vi "FPGA tester without DG535 settings.vi"() -> ()   [LabVIEW 2013]
uses:
  <vilib>/DAQmx/write.llb/DAQmx Write (Digital Bool 1Line 1Point).vi
  <vilib>/DAQmx/read.llb/DAQmx Read (Digital Bool 1Line 1Point).vi
  <vilib>/Utility/file.llb/Read From Spreadsheet File (I64).vi
  <vilib>/DAQmx/miscellaneous.llb/DAQmx Fill In Error Info.vi
panel:
  in  "Delay":u32
  out "Error out":errorcluster[][](array[cluster])
  in  "error in":errorcluster
  out "all rows":i64[][](array[numeric])
  in  "Read Excel file?":bool
  out "Current level":u16
  in  "Repetitions":dbl=1.0
  in  "Levels":i16[](array[numeric])
  out "Set 1":bool[](array[boolean])
  out "Set 2":bool[](array[boolean])
  out "Set 3":bool[](array[boolean])
  out "Set 4":bool[](array[boolean])
  out "16-bit number":bool[](array[boolean])
  # "Or specify levels below:"
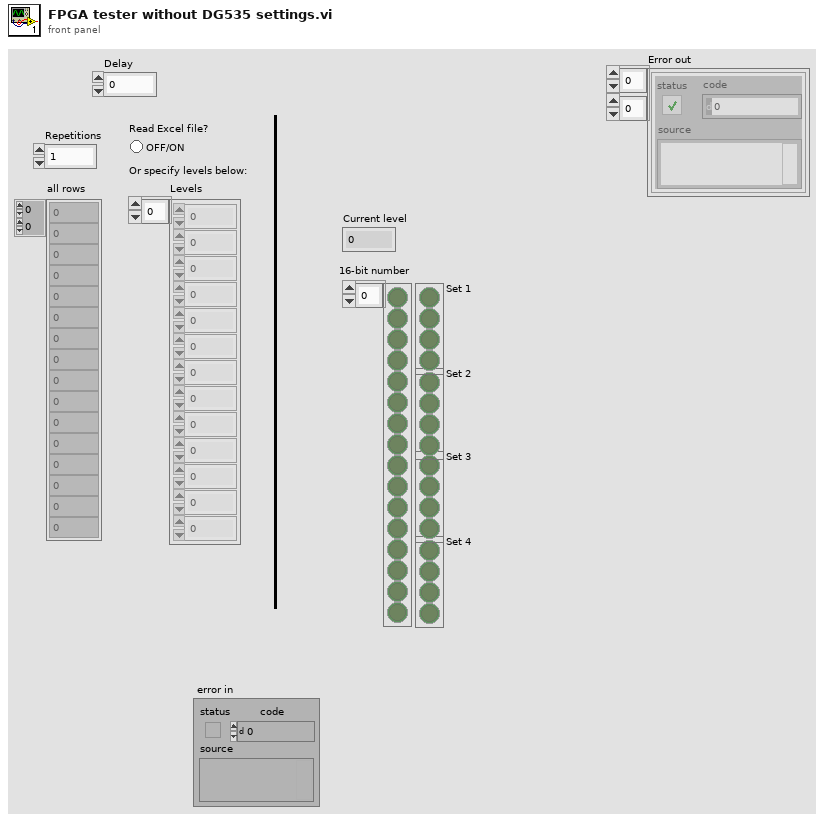
[diagram p1: front panel]
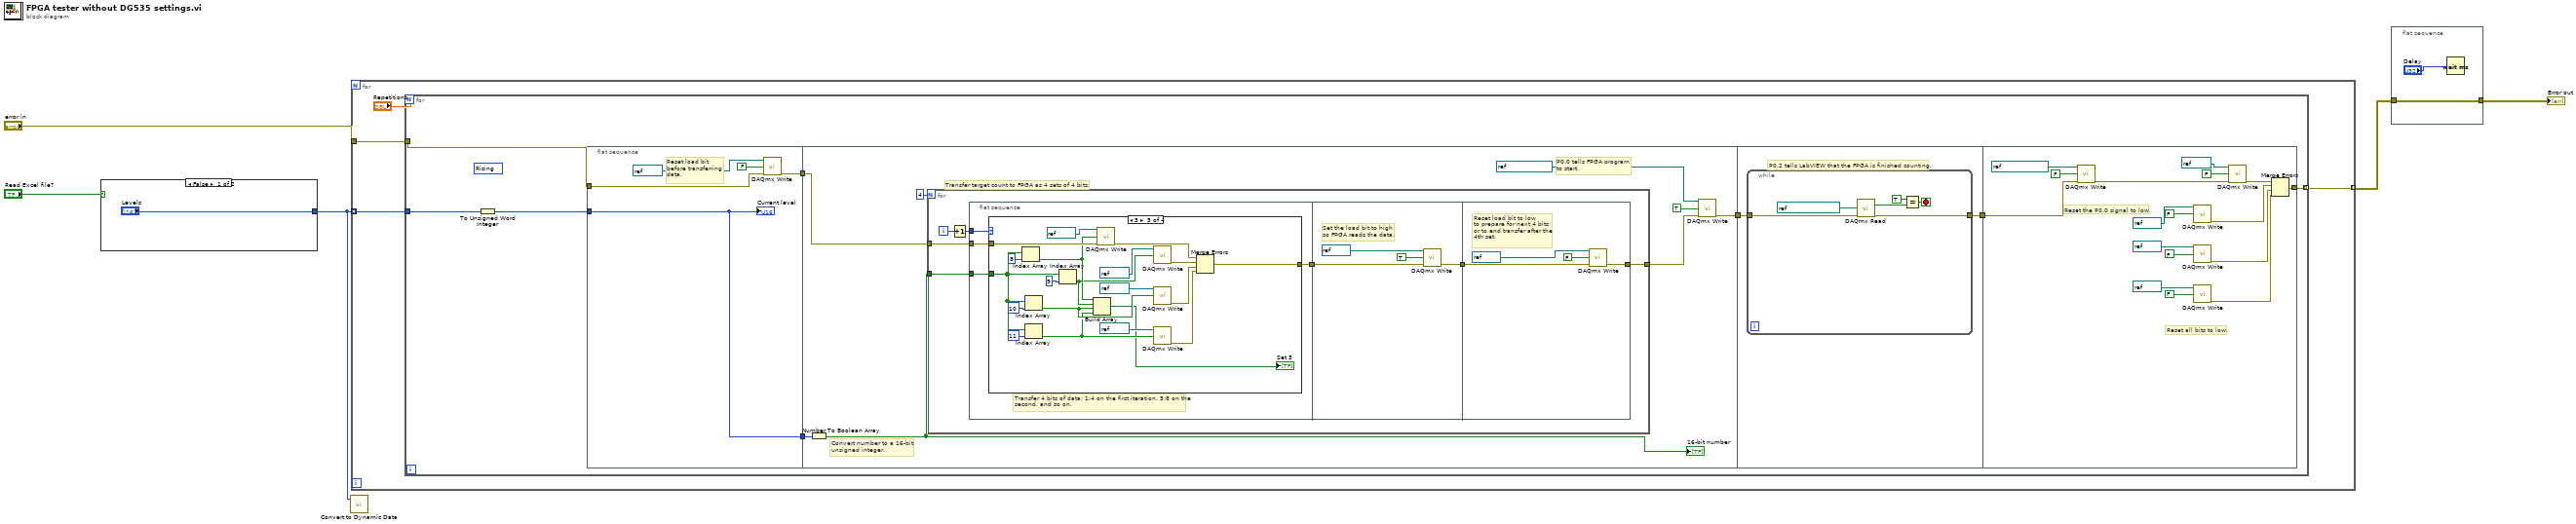
[diagram p0: block diagram]
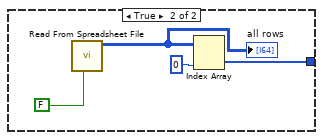
[diagram p2: hidden frame]
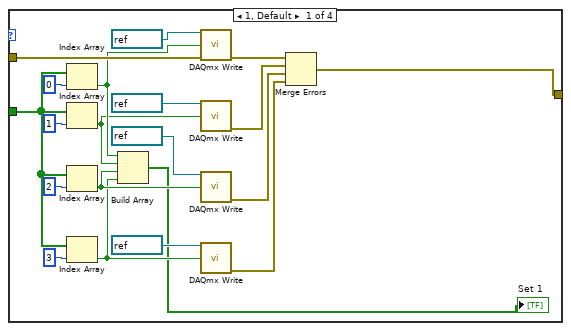
[diagram p3: hidden frame]
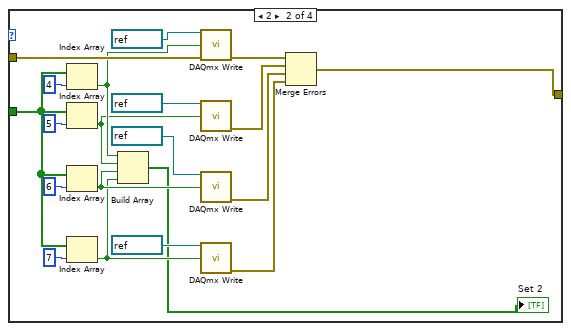
[diagram p4: hidden frame]
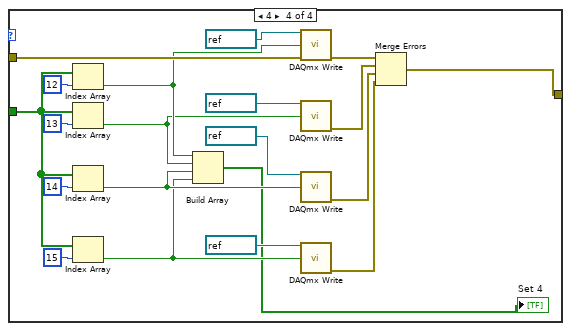
[diagram p5: hidden frame]
diagram:
  n1 = case shown="False" "Read Excel file?" {
    tunnel: ["Levels" w9] -> w4
    frame False {
    }
    frame True {
      n2 = call-poly <vilib>:"Read From Spreadsheet File.vi"("transpose (no:F)"=FALSE) -> ("all rows"=w10:i64[][])  [unwired: 6 in, 4 out]
      "all rows" <- w10
      n3 = Index Array(array=w10, index (col)=0 ("disabled index (col)")) -> (element=w9:i64[])  [unwired: 1 in]
    }
  }
  n4 = call "Convert to Dynamic Data"("Array"=w4) -> ()  [unwired: 3 in, 1 out]
  n5 = for {
    tunnel: w4 -> [w13] mode=indexing
    tunnel: "error in" -> [w12]
    tunnel: [w11] -> w2 mode=indexing
    n6 = for {
      N: "Repetitions" -> [_]
      tunnel: w13 -> [w17]
      tunnel: w12 -> [w15]
      tunnel: [w16] -> w11 mode=indexing
      (unwired) 10280 items=["Rising"=10280, "Falling"=10171] ("Starting Edge")
      n7 = To Unsigned Word Integer(number=w17) -> (unsigned 16bit integer=w18:u16)
      n8 = flat-sequence {
        tunnel: w15 -> [w24]
        tunnel: w18 -> [w27]
        tunnel: [w27] -> w22
        tunnel: [w23] -> w21
        tunnel: [w28] -> w20
        tunnel: w22 -> [w35]
        tunnel: w21 -> [w32]
        tunnel: w20 -> [w136]
        tunnel: [w135] -> w19
        tunnel: [w143] -> w16
        tunnel: w19 -> [w149]
        frame #0 {
          # "Reset load bit\nbefore transferring\ndata."
          n9 = call-poly <vilib>:"DAQmx Write.vi"("task/channels in"=refnum<k21> "BIT5", "data"=FALSE, "error in"=w24) -> ("error out"=w23:errorcluster)  [unwired: 10 in, 2 out]
          "Current level" <- w27
        }
        frame #1 {
          # "P0.0 tells FPGA program \nto start."
          # "Convert number to a 16-bit\nunsigned integer."
          # "Transfer target count to FPGA as 4 sets of 4 bits."
          n10 = Number To Boolean Array(number=w35) -> (Boolean array=w33:bool[])
          "16-bit number" <- w33
          n11 = for {
            N: 4 -> [_]
            tunnel: w33 -> [w39]
            tunnel: w32 -> [w41]
            tunnel: [w36] -> w29
            i -> [w42]
            n12 = Increment(x=w42) -> (x+1=w40:i32)
            n13 = flat-sequence {
              tunnel: w41 -> [w46]
              tunnel: w40 -> [w45]
              tunnel: w39 -> [w44]
              tunnel: [w43] -> w38
              tunnel: w38 -> [w128]
              tunnel: [w127] -> w37
              tunnel: w37 -> [w132]
              tunnel: [w131] -> w36
              frame #0 {
                # "Transfer 4 bits of data: 1:4 on the first iteration, 5:8 on the\nsecond, and so on."
                n14 = case shown="3" w45 {
                  tunnel: w44 -> [w54 w74 w94 w114]
                  tunnel: w46 -> [w53 w73 w93 w113]
                  tunnel: [w52 w72 w92 w112] -> w43
                  frame 1, Default {
                    n15 = Index Array(array=w54, index=0) -> (element=w51:bool)
                    n16 = Index Array(array=w54, index=1) -> (element=w50:bool)
                    n17 = Index Array(array=w54, index=2) -> (element=w49:bool)
                    n18 = Index Array(array=w54, index=3) -> (element=w48:bool)
                    n19 = Build Array(w51, w50, w49, w48) -> (→"Set 1":bool[])
                    n20 = call-poly <vilib>:"DAQmx Write.vi"("task/channels in"=refnum<k21> "BIT1", "data"=w51, "error in"=w53) -> ("error out"=w62:errorcluster)  [unwired: 10 in, 2 out]
                    n21 = call-poly <vilib>:"DAQmx Write.vi"("task/channels in"=refnum<k21> "BIT2", "data"=w50) -> ("error out"=w61:errorcluster)  [unwired: 11 in, 2 out]
                    n22 = call-poly <vilib>:"DAQmx Write.vi"("task/channels in"=refnum<k21> "BIT3", "data"=w49) -> ("error out"=w60:errorcluster)  [unwired: 11 in, 2 out]
                    n23 = call-poly <vilib>:"DAQmx Write.vi"("task/channels in"=refnum<k21> "BIT4", "data"=w48) -> ("error out"=w59:errorcluster)  [unwired: 11 in, 2 out]
                    n24 = Merge Errors(w62, w61, w60, w59) -> (w52:errorcluster)
                  }
                  frame 2 {
                    n25 = Index Array(array=w74, index=4) -> (element=w71:bool)
                    n26 = Index Array(array=w74, index=5) -> (element=w70:bool)
                    n27 = Index Array(array=w74, index=6) -> (element=w69:bool)
                    n28 = Index Array(array=w74, index=7) -> (element=w68:bool)
                    n29 = Build Array(w71, w70, w69, w68) -> (→"Set 2":bool[])
                    n30 = call-poly <vilib>:"DAQmx Write.vi"("task/channels in"=refnum<k21> "BIT1", "data"=w71, "error in"=w73) -> ("error out"=w82:errorcluster)  [unwired: 10 in, 2 out]
                    n31 = call-poly <vilib>:"DAQmx Write.vi"("task/channels in"=refnum<k21> "BIT2", "data"=w70) -> ("error out"=w81:errorcluster)  [unwired: 11 in, 2 out]
                    n32 = call-poly <vilib>:"DAQmx Write.vi"("task/channels in"=refnum<k21> "BIT3", "data"=w69) -> ("error out"=w80:errorcluster)  [unwired: 11 in, 2 out]
                    n33 = call-poly <vilib>:"DAQmx Write.vi"("task/channels in"=refnum<k21> "BIT4", "data"=w68) -> ("error out"=w79:errorcluster)  [unwired: 11 in, 2 out]
                    n34 = Merge Errors(w82, w81, w80, w79) -> (w72:errorcluster)
                  }
                  frame 3 {
                    n35 = Index Array(array=w94, index=8) -> (element=w91:bool)
                    n36 = Index Array(array=w94, index=10) -> (element=w89:bool)
                    n37 = Index Array(array=w94, index=11) -> (element=w88:bool)
                    n38 = Index Array(array=w94, index=9) -> (element=w90:bool)
                    n39 = Build Array(w91, w90, w89, w88) -> (→"Set 3":bool[])
                    n40 = call-poly <vilib>:"DAQmx Write.vi"("task/channels in"=refnum<k21> "BIT1", "data"=w91, "error in"=w93) -> ("error out"=w102:errorcluster)  [unwired: 10 in, 2 out]
                    n41 = call-poly <vilib>:"DAQmx Write.vi"("task/channels in"=refnum<k21> "BIT2", "data"=w90) -> ("error out"=w101:errorcluster)  [unwired: 11 in, 2 out]
                    n42 = call-poly <vilib>:"DAQmx Write.vi"("task/channels in"=refnum<k21> "BIT3", "data"=w89) -> ("error out"=w100:errorcluster)  [unwired: 11 in, 2 out]
                    n43 = call-poly <vilib>:"DAQmx Write.vi"("task/channels in"=refnum<k21> "BIT4", "data"=w88) -> ("error out"=w99:errorcluster)  [unwired: 11 in, 2 out]
                    n44 = Merge Errors(w102, w101, w100, w99) -> (w92:errorcluster)
                  }
                  frame 4 {
                    n45 = Index Array(array=w114, index=12) -> (element=w111:bool)
                    n46 = Index Array(array=w114, index=13) -> (element=w110:bool)
                    n47 = Index Array(array=w114, index=14) -> (element=w109:bool)
                    n48 = Index Array(array=w114, index=15) -> (element=w108:bool)
                    n49 = Build Array(w111, w110, w109, w108) -> (→"Set 4":bool[])
                    n50 = call-poly <vilib>:"DAQmx Write.vi"("task/channels in"=refnum<k21> "BIT1", "data"=w111, "error in"=w113) -> ("error out"=w122:errorcluster)  [unwired: 10 in, 2 out]
                    n51 = call-poly <vilib>:"DAQmx Write.vi"("task/channels in"=refnum<k21> "BIT2", "data"=w110) -> ("error out"=w121:errorcluster)  [unwired: 11 in, 2 out]
                    n52 = call-poly <vilib>:"DAQmx Write.vi"("task/channels in"=refnum<k21> "BIT3", "data"=w109) -> ("error out"=w120:errorcluster)  [unwired: 11 in, 2 out]
                    n53 = call-poly <vilib>:"DAQmx Write.vi"("task/channels in"=refnum<k21> "BIT4", "data"=w108) -> ("error out"=w119:errorcluster)  [unwired: 11 in, 2 out]
                    n54 = Merge Errors(w122, w121, w120, w119) -> (w112:errorcluster)
                  }
                }
              }
              frame #1 {
                # "Set the load bit to high\nso FPGA reads the data."
                n55 = call-poly <vilib>:"DAQmx Write.vi"("task/channels in"=refnum<k21> "BIT5", "data"=TRUE, "error in"=w128) -> ("error out"=w127:errorcluster)  [unwired: 10 in, 2 out]
              }
              frame #2 {
                # "Reset load bit to low\nto prepare for next 4 bits\nor to end transfer after the\n4th set."
                n56 = call-poly <vilib>:"DAQmx Write.vi"("task/channels in"=refnum<k21> "BIT5", "data"=FALSE, "error in"=w132) -> ("error out"=w131:errorcluster)  [unwired: 10 in, 2 out]
              }
            }
          }
          n57 = call-poly <vilib>:"DAQmx Write.vi"("task/channels in"=refnum<k21> "LaserChannel", "data"=TRUE, "error in"=w29) -> ("error out"=w28:errorcluster)  [unwired: 10 in, 2 out]
        }
        frame #2 {
          # "P0.2 tells LabVIEW that the FPGA is finished counting."
          n58 = while {
            tunnel: w136 -> [w142]
            tunnel: [w141] -> w135
            stop <- w138 stop-if-true
            n59 = call-poly <vilib>:"DAQmx Read.vi"("task/channels in"=refnum<k21> "P02countSignal", "error in"=w142) -> ("data"=w139:bool, "error out"=w141:errorcluster)  [unwired: 11 in, 1 out]
            n60 = Equal?(x=TRUE, y=w139) -> (x = y?=w138:bool)
          }
        }
        frame #3 {
          # "Reset all bits to low."
          # "Reset the P0.0 signal to low."
          n61 = call-poly <vilib>:"DAQmx Write.vi"("task/channels in"=refnum<k21> "LaserChannel", "data"=FALSE, "error in"=w149) -> ("error out"=w148:errorcluster)  [unwired: 10 in, 2 out]
          n62 = call-poly <vilib>:"DAQmx Write.vi"("task/channels in"=refnum<k21> "BIT2", "data"=FALSE) -> ("error out"=w156:errorcluster)  [unwired: 11 in, 2 out]
          n63 = call-poly <vilib>:"DAQmx Write.vi"("task/channels in"=refnum<k21> "BIT3", "data"=FALSE) -> ("error out"=w155:errorcluster)  [unwired: 11 in, 2 out]
          n64 = call-poly <vilib>:"DAQmx Write.vi"("task/channels in"=refnum<k21> "BIT4", "data"=FALSE) -> ("error out"=w154:errorcluster)  [unwired: 11 in, 2 out]
          n65 = call-poly <vilib>:"DAQmx Write.vi"("task/channels in"=refnum<k21> "BIT1", "data"=FALSE, "error in"=w148) -> ("error out"=w157:errorcluster)  [unwired: 10 in, 2 out]
          n66 = Merge Errors(w157, w156, w155, w154) -> (w143:errorcluster)
        }
      }
    }
  }
  n67 = flat-sequence {
    tunnel: w2 -> [w161]
    tunnel: [w161] -> w1
    frame #0 {
      n68 = Wait (ms)(milliseconds to wait="Delay") -> ()  [unwired: 1 out]
    }
  }
  "Error out" <- w1
